vi "读取摄像头.vi"(8 "error  in":errorcluster, 9 "Image In":T1, 10 "Boolean":bool, 11 "Session in":T2) -> (0 "error out":errorcluster, 1 "Image Out":T1, 2 "Session Out 2":T2)   [LabVIEW 2015]
uses:
  <vilib>/userdefined/High Color/IMAQdx.ctl
  <vilib>/vision/Image Controls.llb/IMAQ Image.ctl
  <vilib>/vision/driver/NI_Vision_Acquisition_Software.lvlib
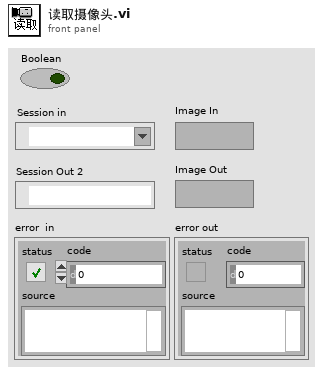
[diagram p1: front panel]
types:
  T1 = typedef "IMAQ Image.ctl" = refnum<image>
  T2 = typedef "IMAQdx.ctl" = refnum<k21>
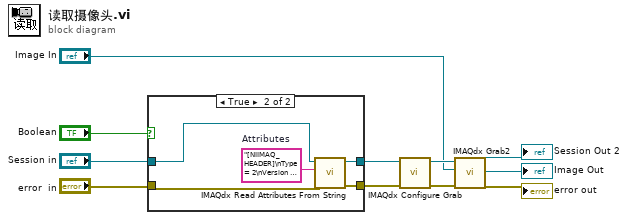
[diagram p0: block diagram]
diagram:
  n1 = case shown="True" "Boolean" {
    tunnel: "Session in" -> [w13 w18]
    tunnel: "error  in" -> [w12 w16]
    tunnel: [w13 w15] -> w11
    tunnel: [w12 w14] -> w9
    frame False {
    }
    frame True {
      w17 = "[NIIMAQ_HEADER]\nType = 2\nVersion = 8\n\n[CAMERA_DATA]\nAcquisitionAttributes::Bayer::Algorithm = \"Bilinear\"\nAcquisitionAttributes::Bayer::GainB = \"1\"\nAcquisitionAttributes::Bayer::GainG = \"1\"\nAcquisitionAttributes::Bayer::GainR = \"1\"\nAcquisitionAttributes::Bayer::Pattern = \"Use hardware value\"\nAcquisitionAttributes::BitsPerPixel = \"Use hardware value\"\nAcquisitionAttributes::IgnoreFirstFrame = \"false\"\nAcquisitionAttributes::ImageDecoderCopyMode = \"Auto\"\nAcquisitionAttributes::OutputImageType = \"Auto\"\nAcquisitionAttributes::OverwriteMode = \"Get Newest\"\nAcquisitionAttributes::PixelSignedness = \"Use hardware value\"\nAcquisitionAttributes::ReceiveTimestampMode = \"None\"\nAcquisitionAttributes::ShiftPixelBits = \"false\"\nAcquisitionAttributes::SwapPixelBytes = \"false\"\nAcquisitionAttributes::Timeout = \"5000\"\nAcquisitionAttributes::VideoMode = \"640 x 480 JPEG 20.00 fps\"\nCameraAttributes::BacklightCompensation::Mode = \"Manual\"\nCameraAttributes::BacklightCompensation::Value = \"1\"\nCameraAttributes::Brightness::Mode = \"Manual\"\nCameraAttributes::Brightness::Value = \"0\"\nCameraAttributes::Contrast::Mode = \"Manual\"\nCameraAttributes::Contrast::Value = \"36\"\nCameraAttributes::Exposure::Mode = \"AutoAperaturePriority\"\nCameraAttributes::Gain::Mode = \"Manual\"\nCameraAttributes::Gain::Value = \"0\"\nCameraAttributes::Gamma::Mode = \"Manual\"\nCameraAttributes::Gamma::Value = \"100\"\nCameraAttributes::Hue::Mode = \"Manual\"\nCameraAttributes::Hue::Value = \"0\"\nCameraAttributes::PowerLineFrequency::Mode = \"50Hz\"\nCameraAttributes::Saturation::Mode = \"Manual\"\nCameraAttributes::Saturation::Value = \"0\"\nCameraAttributes::Sharpness::Mode = \"Manual\"\nCameraAttributes::Sharpness::Value = \"1\"\nCameraAttributes::WhiteBalance::Mode = \"Auto\"\n"  # Attributes
      n2 = call <vilib>:"IMAQdx Read Attributes From String.vi"("error in"=w16, "Attributes String In"=w17, "Session In"=w18) -> ("error out"=w14:errorcluster, "Session Out"=w15:T2)  [unwired: 7 out]
    }
  }
  n3 = call <vilib>:"IMAQdx Configure Grab.vi"("error in"=w9, "Session In"=w11) -> ("error out"=w8:errorcluster, "Session Out"=w10:T2)  [unwired: 8 out]
  n4 = call <vilib>:"IMAQdx Grab2.vi"("error in"=w8, "Image In"="Image In", "Session In"=w10) -> ("error out"=→"error out":errorcluster, "Image Out"=→"Image Out":T1, "Session Out"=→"Session Out 2":T2)  [unwired: 5 in, 1 out]
